vi "Thermistor_Callibration.vi"(11 "DataCluster in":T2={"Core"={"Current VI Reference"=refnum, "Close Panel on Exit?"=FALSE, "Exit"=FALSE, "Initialized?"=FALSE}, "Connections"={"cDAQ"={"Task"="", "Connected"=FALSE, "Active"=FALSE, "ID"=""}, "Camera"={"Session"="", "Connected"=FALSE, "Active"=FALSE, "Placeholder"=refnum}, "PSU"={"Port"="", "Connected"=FALSE, "Active"=FALSE}, "Arduino"={"Port"="", "Connected"=FALSE, "Active"=FALSE}}, "Data Acquisition"={"Setup"={"Label"="", "Operator"="", "Notes"="", "TempGrad"=1.0, "TargetTemp"=1.0, "Sample Volume"=1.0}, "Camera"={"Image"=refnum, "Save Image"=refnum, "Image Frequency"=20, "Rectangle"={"Left"=0, "Top"=0, "Right"=0, "Bottom"=0, "Rotation"=0.0}, "Calibration"={"Top Left"={"X"=0.0, "Y"=0.0}, "Top Right"={"X"=0.0, "Y"=0.0}, "Bottom Left"={"X"=0.0, "Y"=0.0}, "Bottom Right"={"X"=0.0, "Y"=0.0}, "Fixpoint"={"X"=0.0, "Y"=0.0}, "Scan Area"=0.0, "Fixpoint Area"=0.0, "Well Pixels"=[], "Valid"=FALSE}, "FocusPos"=0, "Display Mapping"=10, "Camera Mode"=10}, "Thermistor"={"Sample Size"=1, "Calibration"={"B0.100"=[], "R25"=[], "c"=[], "State"=[], "V_S"=5.0, "R_S"=100.0}, "Timing Mode"=14713}, "Partition"={"Data"=[], "Cell Label"="", "Cell Color"=0, "Height"=10, "Width"=16, "Grid"=[]}, "Queue"={"Size"=1, "Queue"=refnum}, "Sample Rate"=1, "Active"=FALSE, "Ready"=FALSE, "Graph Mode"=0, "Gradient Buffer"=2}, "Control"={"Sample Rate"=1, "PID gains"={"proportional gain (Kc)"=1.0, "integral time (Ti, min)"=0.01, "derivative time (Td, min)"=0.0}}, "Manual Temp Control"={"TargetTemp"=1.0, "Mode"=0, "Active"=FALSE}} {"Manual Temp Control"."Mode" items=["Cool", "Heat"]; "Manual Temp Control"."TargetTemp" min=-40.0 max=40.0 step=0.5 format="%#_g °C"; "Control"."PID gains"."derivative time (Td, min)" format="%.3f"; "Control"."PID gains"."integral time (Ti, min)" format="%.3f"; "Control"."PID gains"."proportional gain (Kc)" format="%.3f"; "Control"."Sample Rate" min=1 max=20 step=1 format="%.0f Samples/sec"; "Data Acquisition"."Gradient Buffer" min=2 max=30 step=1; "Data Acquisition"."Graph Mode" items=["Thermistor Temperature", "Camera Temperature"]; "Data Acquisition"."Thermistor"."Timing Mode" items=["Automatic"=16097, "High Resolution"=10195, "High Speed"=14712, "Best 50 Hz Rejection"=14713, "Best 60 Hz Rejection"=14714, "Custom"=10137]; "Data Acquisition"."Thermistor"."Calibration"."R_S" min=0.1 max=1000.0 format="%#_g kOhm"; "Data Acquisition"."Thermistor"."Calibration"."V_S" min=5.0 max=48.0 format="%#_g V"; "Data Acquisition"."Thermistor"."Calibration"."R25" min=0.1 max=1000.0 format="%#_g kOhm"; "Data Acquisition"."Thermistor"."Calibration"."B0.100" min=100.0 max=10000.0 format="%#_g K"; "Data Acquisition"."Thermistor"."Sample Size" min=1 max=200; "Data Acquisition"."Sample Rate" min=20 max=240 format="%.0f samples/min"; "Data Acquisition"."Queue"."Size" min=1 max=200; "Data Acquisition"."Camera"."Camera Mode" items=["Temperature Linear", "Signal Linear"]; "Data Acquisition"."Camera"."Display Mapping" items=["Default"=10, "Most Significant Bits"=11, "Full Dynamic"=12, "Downshift"=13, "Given Range"=14, "90% Dynamic"=15, "Given Percent Range"=16]; "Data Acquisition"."Camera"."Calibration"."Fixpoint"."Y" format="%.2f"; "Data Acquisition"."Camera"."Calibration"."Fixpoint"."X" format="%.2f"; "Data Acquisition"."Camera"."Calibration"."Top Left"."Y" format="%.2f"; "Data Acquisition"."Camera"."Calibration"."Top Left"."X" format="%.2f"; "Data Acquisition"."Camera"."Calibration"."Top Right"."Y" format="%.2f"; "Data Acquisition"."Camera"."Calibration"."Top Right"."X" format="%.2f"; "Data Acquisition"."Camera"."Calibration"."Bottom Left"."Y" format="%.2f"; "Data Acquisition"."Camera"."Calibration"."Bottom Left"."X" format="%.2f"; "Data Acquisition"."Camera"."Calibration"."Bottom Right"."Y" format="%.2f"; "Data Acquisition"."Camera"."Calibration"."Bottom Right"."X" format="%.2f"; "Data Acquisition"."Camera"."Rectangle"."Rotation" min=-90.0 max=90.0 step=1.0 format="%.2f"; "Data Acquisition"."Camera"."Rectangle"."Left" scale=0.0..1024.0; "Data Acquisition"."Camera"."Rectangle"."Right" scale=0.0..1024.0; "Data Acquisition"."Camera"."Image Frequency" min=1 max=60 step=1; "Data Acquisition"."Setup"."Sample Volume" min=0.0 max=500.0 format="%#_g µL"; "Data Acquisition"."Setup"."TargetTemp" min=-40.0 max=40.0 step=0.5 format="%#_g °C"; "Data Acquisition"."Setup"."TempGrad" min=-100.0 max=100.0 step=0.1 format="%#_g °C/min"}) -> (2 "State Out":string="Data: Save Calibration", 3 "DataCluster out":T2={"Core"={"Current VI Reference"=refnum, "Close Panel on Exit?"=FALSE, "Exit"=FALSE, "Initialized?"=FALSE}, "Connections"={"cDAQ"={"Task"="", "Connected"=FALSE, "Active"=FALSE, "ID"=""}, "Camera"={"Session"="", "Connected"=FALSE, "Active"=FALSE, "Placeholder"=refnum}, "PSU"={"Port"="", "Connected"=FALSE, "Active"=FALSE}, "Arduino"={"Port"="", "Connected"=FALSE, "Active"=FALSE}}, "Data Acquisition"={"Setup"={"Label"="", "Operator"="", "Notes"="", "TempGrad"=0.0, "TargetTemp"=0.0, "Sample Volume"=0.0}, "Camera"={"Image"=refnum, "Save Image"=refnum, "Image Frequency"=20, "Rectangle"={"Left"=0, "Top"=0, "Right"=0, "Bottom"=0, "Rotation"=0.0}, "Calibration"={"Top Left"={"X"=0.0, "Y"=0.0}, "Top Right"={"X"=0.0, "Y"=0.0}, "Bottom Left"={"X"=0.0, "Y"=0.0}, "Bottom Right"={"X"=0.0, "Y"=0.0}, "Fixpoint"={"X"=0.0, "Y"=0.0}, "Scan Area"=0.0, "Fixpoint Area"=0.0, "Well Pixels"=[], "Valid"=FALSE}, "FocusPos"=0, "Display Mapping"=10, "Camera Mode"=10}, "Thermistor"={"Sample Size"=0, "Calibration"={"B0.100"=[], "R25"=[], "c"=[], "State"=[], "V_S"=0.0, "R_S"=0.0}, "Timing Mode"=0}, "Partition"={"Data"=[], "Cell Label"="", "Cell Color"=0, "Height"=0, "Width"=0, "Grid"=[]}, "Queue"={"Size"=0, "Queue"=refnum}, "Sample Rate"=0, "Active"=FALSE, "Ready"=FALSE, "Graph Mode"=0, "Gradient Buffer"=2}, "Control"={"Sample Rate"=0, "PID gains"={"proportional gain (Kc)"=0.0, "integral time (Ti, min)"=0.0, "derivative time (Td, min)"=0.0}}, "Manual Temp Control"={"TargetTemp"=1.0, "Mode"=0, "Active"=FALSE}} {"Manual Temp Control"."Mode" items=["Cool", "Heat"]; "Manual Temp Control"."TargetTemp" min=-40.0 max=40.0 step=0.5 format="%#_g °C"; "Control"."PID gains"."derivative time (Td, min)" format="%.3f"; "Control"."PID gains"."integral time (Ti, min)" format="%.3f"; "Control"."PID gains"."proportional gain (Kc)" format="%.3f"; "Control"."Sample Rate" min=1 max=20 step=1 format="%.0f Samples/sec"; "Data Acquisition"."Gradient Buffer" min=2 max=30 step=1; "Data Acquisition"."Graph Mode" items=["Thermistor Temperature", "Camera Temperature"]; "Data Acquisition"."Thermistor"."Timing Mode" items=["Automatic"=16097, "High Resolution"=10195, "High Speed"=14712, "Best 50 Hz Rejection"=14713, "Best 60 Hz Rejection"=14714, "Custom"=10137]; "Data Acquisition"."Thermistor"."Calibration"."R_S" min=0.1 max=1000.0 format="%#_g kOhm"; "Data Acquisition"."Thermistor"."Calibration"."V_S" min=5.0 max=48.0 format="%#_g V"; "Data Acquisition"."Thermistor"."Calibration"."R25" min=0.1 max=1000.0 format="%#_g kOhm"; "Data Acquisition"."Thermistor"."Calibration"."B0.100" min=100.0 max=10000.0 format="%#_g K"; "Data Acquisition"."Thermistor"."Sample Size" min=1 max=200; "Data Acquisition"."Sample Rate" min=20 max=240 format="%.0f samples/min"; "Data Acquisition"."Queue"."Size" min=1 max=200; "Data Acquisition"."Camera"."Camera Mode" items=["Temperature Linear", "Signal Linear"]; "Data Acquisition"."Camera"."Display Mapping" items=["Default"=10, "Most Significant Bits"=11, "Full Dynamic"=12, "Downshift"=13, "Given Range"=14, "90% Dynamic"=15, "Given Percent Range"=16]; "Data Acquisition"."Camera"."Calibration"."Fixpoint"."Y" format="%.2f"; "Data Acquisition"."Camera"."Calibration"."Fixpoint"."X" format="%.2f"; "Data Acquisition"."Camera"."Calibration"."Top Left"."Y" format="%.2f"; "Data Acquisition"."Camera"."Calibration"."Top Left"."X" format="%.2f"; "Data Acquisition"."Camera"."Calibration"."Top Right"."Y" format="%.2f"; "Data Acquisition"."Camera"."Calibration"."Top Right"."X" format="%.2f"; "Data Acquisition"."Camera"."Calibration"."Bottom Left"."Y" format="%.2f"; "Data Acquisition"."Camera"."Calibration"."Bottom Left"."X" format="%.2f"; "Data Acquisition"."Camera"."Calibration"."Bottom Right"."Y" format="%.2f"; "Data Acquisition"."Camera"."Calibration"."Bottom Right"."X" format="%.2f"; "Data Acquisition"."Camera"."Rectangle"."Rotation" min=-90.0 max=90.0 step=1.0 format="%.2f"; "Data Acquisition"."Camera"."Rectangle"."Left" scale=0.0..1024.0; "Data Acquisition"."Camera"."Rectangle"."Right" scale=0.0..1024.0; "Data Acquisition"."Camera"."Image Frequency" min=1 max=60 step=1; "Data Acquisition"."Setup"."Sample Volume" min=0.0 max=500.0 format="%#_g µL"; "Data Acquisition"."Setup"."TargetTemp" min=-40.0 max=40.0 step=0.5 format="%#_g °C"; "Data Acquisition"."Setup"."TempGrad" min=-100.0 max=100.0 step=0.1 format="%#_g °C/min"})   [LabVIEW 2024]
uses:
  DataCluster.ctl
  <vilib>/userDefined/High Color/IMAQdx.ctl
  <vilib>/vision/Image Controls.llb/IMAQ Image.ctl
panel:
  in  "Ring":u16(ring) items=["Setup", "Thermistor (Ref.)", "Thermistor 1", "Thermistor 2", "Thermistor 3", "Thermistor 4", "Thermistor 5", "Thermistor 6"]
  out "Tab Control":T1(tab)
  in  "Supply Voltage":dbl=12.062 format="%#_g V"
  in  "Static Resistor":dbl=10.0 min=0.1 max=1000.0 format="%#_g kOhm"
  out "Active":bool
  in  "c ref":dbl[](array[numeric]) caption="constants" format="%_6g"
  in  "B0.100 ref":dbl caption="ß0.100" min=0.0 format="%#_g K"
  in  "R25 ref":dbl caption="R25" min=0.0 format="%#_g kOhm"
  in  "Active 1":bool
  in  "B0.100 1":dbl caption="ß0.100" min=0.0 format="%#_g K"
  in  "R25 1":dbl caption="R25" min=0.0 format="%#_g kOhm"
  in  "c 1":dbl[](array[numeric]) caption="constants" format="%_6g"
  in  "Active 2":bool
  in  "B0.100 2":dbl caption="ß0.100" min=0.0 format="%#_g K"
  in  "R25 2":dbl caption="R25" min=0.0 format="%#_g kOhm"
  in  "c 2":dbl[](array[numeric]) caption="constants" format="%_6g"
  in  "Active 3":bool
  in  "B0.100 3":dbl caption="ß0.100" min=0.0 format="%#_g K"
  in  "R25 3":dbl caption="R25" min=0.0 format="%#_g kOhm"
  in  "c 3":dbl[](array[numeric]) caption="constants" format="%_6g"
  in  "Active 4":bool
  in  "B0.100 4":dbl caption="ß0.100" min=0.0 format="%#_g K"
  in  "R25 4":dbl caption="R25" min=0.0 format="%#_g kOhm"
  in  "c 4":dbl[](array[numeric]) caption="constants" format="%_6g"
  in  "Active 5":bool
  in  "B0.100 5":dbl caption="ß0.100" min=0.0 format="%#_g K"
  in  "R25 5":dbl caption="R25" min=0.0 format="%#_g kOhm"
  in  "c 5":dbl[](array[numeric]) caption="constants" format="%_6g"
  in  "Active 6":bool
  in  "B0.100 6":dbl caption="ß0.100" min=0.0 format="%#_g K"
  in  "R25 6":dbl caption="R25" min=0.0 format="%#_g kOhm"
  in  "c 6":dbl[](array[numeric]) caption="constants" format="%_6g"
  in  "Cancel":bool
  in  "OK":bool
  # "Adjust thermistor calibration values used in conversion between measured voltages and temperatures"
  # "c0"
  # "c1"
  # "c2"
  # "c3"
  # "c4"
  # "c0"
  # "c1"
  # "c2"
  # "c3"
  # "c4"
  # "c0"
  # "c1"
  # "c2"
  # "c3"
  # "c4"
  # "c0"
  # "c1"
  # "c2"
  # "c3"
  # "c4"
  # "c0"
  # "c1"
  # "c2"
  # "c3"
  # "c4"
  # "c0"
  # "c1"
  # "c2"
  # "c3"
  # "c4"
  # "c0"
  # "c1"
  # "c2"
  # "c3"
  # "c4"
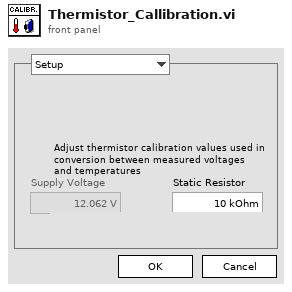
[diagram p1: front panel]
types:
  T1 = enum32{"Setup", "1", "2", "3", "4", "5", "6", "7", "8"}
  T2 = typedef "DataCluster.ctl" = cluster{"Core":cluster{"Current VI Reference":refnum<vi>, "Close Panel on Exit?":bool, "Exit":bool, "Initialized?":bool}, "Connections":cluster{"cDAQ":cluster{"Task":refnum<k21>, "Connected":bool, "Active":bool, "ID":string}, "Camera":cluster{"Session":T3, "Connected":bool, "Active":bool, "Placeholder":T4}, "PSU":cluster{"Port":refnum<visa-resource-name>, "Connected":bool, "Active":bool}, "Arduino":cluster{"Port":refnum<visa-resource-name>, "Connected":bool, "Active":bool}}, "Data Acquisition":cluster{"Setup":cluster{"Label":string, "Operator":string, "Notes":string, "TempGrad":dbl, "TargetTemp":dbl, "Sample Volume":dbl}, "Camera":cluster{"Image":T4, "Save Image":T4, "Image Frequency":i32, "Rectangle":T5, "Calibration":cluster{"Top Left":T6, "Top Right":T6, "Bottom Left":T6, "Bottom Right":T6, "Fixpoint":T6, "Scan Area":dbl, "Fixpoint Area":dbl, "Well Pixels":cluster{"X":i32, "Y":i32}[][], "Valid":bool}, "FocusPos":u32, "Display Mapping":u32, "Camera Mode":u32}, "Thermistor":cluster{"Sample Size":i32, "Calibration":cluster{"B0.100":dbl[], "R25":dbl[], "c":dbl[][], "State":bool[], "V_S":dbl, "R_S":dbl}, "Timing Mode":i32}, "Partition":cluster{"Data":string[][], "Cell Label":string, "Cell Color":u32, "Height":i32, "Width":i32, "Grid":string[][]}, "Queue":cluster{"Size":i32, "Queue":refnum<queue>}, "Sample Rate":i32, "Active":bool, "Ready":bool, "Graph Mode":u16, "Gradient Buffer":i32}, "Control":cluster{"Sample Rate":i32, "PID gains":cluster{"proportional gain (Kc)":dbl, "integral time (Ti, min)":dbl, "derivative time (Td, min)":dbl}}, "Manual Temp Control":cluster{"TargetTemp":dbl, "Mode":u16, "Active":bool}}
  T3 = typedef "IMAQdx.ctl" = refnum<k21>
  T4 = typedef "IMAQ Image.ctl" = refnum<image>
  T5 = typedef "IMAQ Rectangle" = cluster{"Left":i32, "Top":i32, "Right":i32, "Bottom":i32, "Rotation":dbl}
  T6 = typedef "IMAQ Point" = cluster{"X":sgl, "Y":sgl}
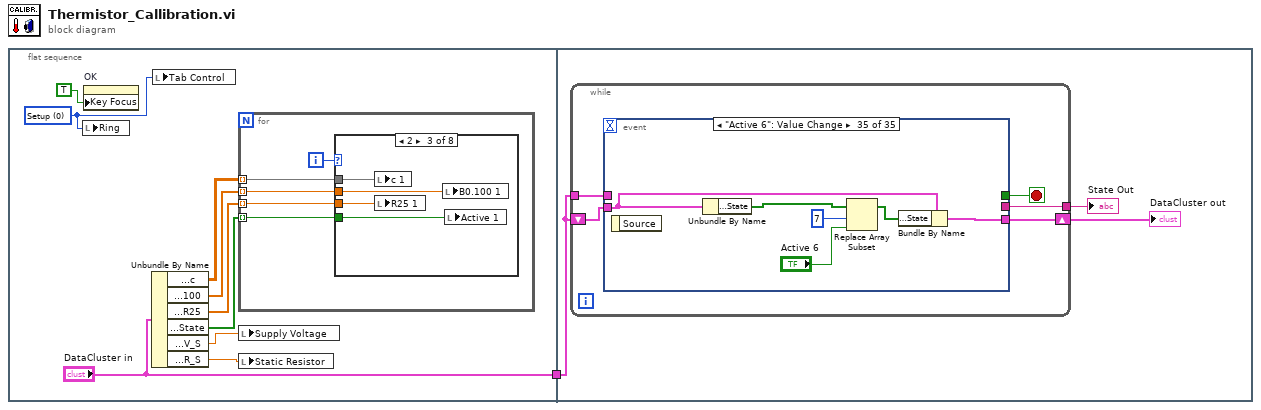
[diagram p0: block diagram]
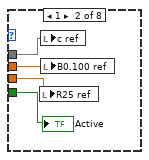
[diagram p3: hidden frame]
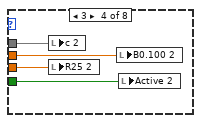
[diagram p4: hidden frame]
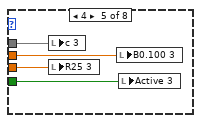
[diagram p5: hidden frame]
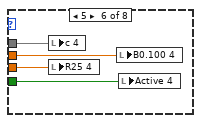
[diagram p6: hidden frame]
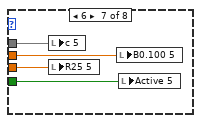
[diagram p7: hidden frame]
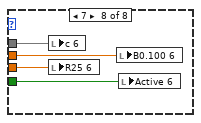
[diagram p8: hidden frame]
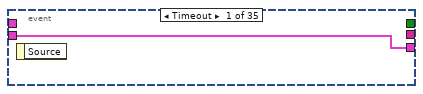
[diagram p9: hidden frame]
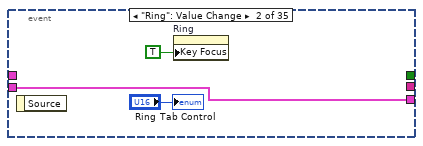
[diagram p10: hidden frame]
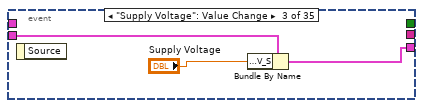
[diagram p11: hidden frame]
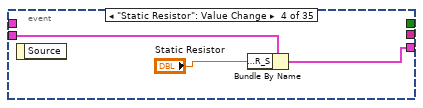
[diagram p12: hidden frame]
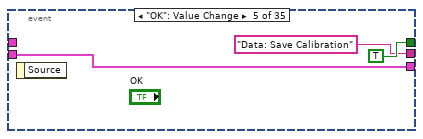
[diagram p13: hidden frame]
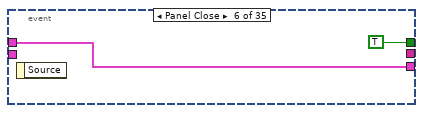
[diagram p14: hidden frame]
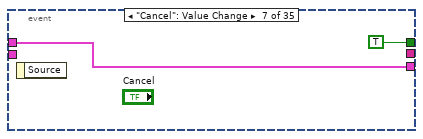
[diagram p15: hidden frame]
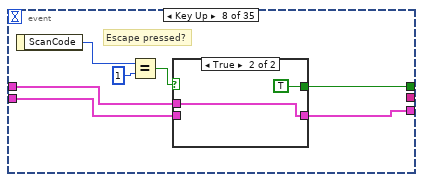
[diagram p16: hidden frame]
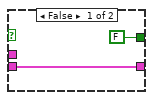
[diagram p17: hidden frame]
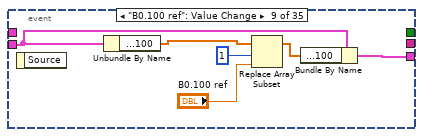
[diagram p18: hidden frame]
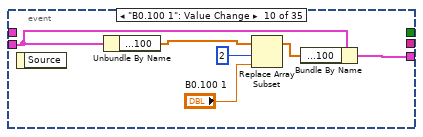
[diagram p19: hidden frame]
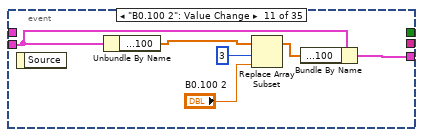
[diagram p20: hidden frame]
diagram:
  n1 = flat-sequence {
    tunnel: ["DataCluster in"] -> w1
    tunnel: w1 -> [w46]
    frame #0 {
      w4 = u16 0 items=["Setup", "Thermistor (Ref.)", "Thermistor 1", "Thermistor 2", "Thermistor 3", "Thermistor 4", "Thermistor 5", "Thermistor 6"] ("Ring")
      n2 = local write "Ring"(w4) -> ()
      n3 = property on="OK" class="Bool"("Key Focus"=TRUE) -> ()  [unwired: 2 in, 2 out]
      n4 = Unbundle By Name("DataCluster in") -> ("Data Acquisition.Thermistor.Calibration.c"=w3:dbl[][], "Data Acquisition.Thermistor.Calibration.B0.100"=w5:dbl[], "Data Acquisition.Thermistor.Calibration.R25"=w6:dbl[], "Data Acquisition.Thermistor.Calibration.State"=w2:bool[], "Data Acquisition.Thermistor.Calibration.V_S"=w8:dbl, "Data Acquisition.Thermistor.Calibration.R_S"=w7:dbl)
      n5 = local write "Tab Control"(w4) -> ()
      n6 = for {
        tunnel: w6 -> [w14] mode=indexing
        tunnel: w5 -> [w13] mode=indexing
        tunnel: w3 -> [w12] mode=indexing
        tunnel: w2 -> [w11] mode=indexing
        i -> [w15]
        n7 = case shown="2" w15 {
          tunnel: w14 -> [_ w19 w23 w27 w31 w35 w39 w43]
          tunnel: w13 -> [_ w18 w22 w26 w30 w34 w38 w42]
          tunnel: w12 -> [_ w17 w21 w25 w29 w33 w37 w41]
          tunnel: w11 -> [_ w16 w20 w24 w28 w32 w36 w40]
          frame 0, Default {
          }
          frame 1 {
            n8 = local write "R25 ref"(w19) -> ()
            n9 = local write "c ref"(w17) -> ()
            n10 = local write "B0.100 ref"(w18) -> ()
            "Active" <- w16
          }
          frame 2 {
            n11 = local write "c 1"(w21) -> ()
            n12 = local write "R25 1"(w23) -> ()
            n13 = local write "B0.100 1"(w22) -> ()
            n14 = local write "Active 1"(w20) -> ()
          }
          frame 3 {
            n15 = local write "c 2"(w25) -> ()
            n16 = local write "R25 2"(w27) -> ()
            n17 = local write "B0.100 2"(w26) -> ()
            n18 = local write "Active 2"(w24) -> ()
          }
          frame 4 {
            n19 = local write "c 3"(w29) -> ()
            n20 = local write "R25 3"(w31) -> ()
            n21 = local write "B0.100 3"(w30) -> ()
            n22 = local write "Active 3"(w28) -> ()
          }
          frame 5 {
            n23 = local write "c 4"(w33) -> ()
            n24 = local write "R25 4"(w35) -> ()
            n25 = local write "B0.100 4"(w34) -> ()
            n26 = local write "Active 4"(w32) -> ()
          }
          frame 6 {
            n27 = local write "c 5"(w37) -> ()
            n28 = local write "R25 5"(w39) -> ()
            n29 = local write "B0.100 5"(w38) -> ()
            n30 = local write "Active 5"(w36) -> ()
          }
          frame 7 {
            n31 = local write "c 6"(w41) -> ()
            n32 = local write "R25 6"(w43) -> ()
            n33 = local write "B0.100 6"(w42) -> ()
            n34 = local write "Active 6"(w40) -> ()
          }
        }
      }
      n35 = local write "Supply Voltage"(w8) -> ()
      n36 = local write "Static Resistor"(w7) -> ()
    }
    frame #1 {
      n37 = while {
        shift-right: [w51] -> w45
        shift-left: w46 -> [w50]
        tunnel: w46 -> [w49]
        tunnel: [w47] -> w44
        stop <- w48 stop-if-true
        n38 = event shown="[34] \"Active 6\": Value Change" {
          selector: _ -> [_ _ _ _ _ _ _ _ _ _ _ _ _ _ _ _ _ _ _ _ _ _ _ _ _ _ _ _ _ _ _ _ _ _ _]
          dyn-events: _ -> [_ _ _ _ _ _ _ _ _ _ _ _ _ _ _ _ _ _ _ _ _ _ _ _ _ _ _ _ _ _ _ _ _ _ _]
          timeout: _ -> [_ _ _ _ _ _ _ _ _ _ _ _ _ _ _ _ _ _ _ _ _ _ _ _ _ _ _ _ _ _ _ _ _ _ _]
          tunnel: w50 -> [w52 w54 w58 w61 w64 _ _ w69 w84 w90 w96 w102 w108 w114 w120 w126 w132 w138 w144 w150 w156 w162 w168 w174 w180 w186 w192 w198 w204 w210 w216 w222 w228 w234 w240]
          tunnel: [w52 w54 w57 w60 w64 w65 w68 w71 w85 w91 w97 w103 w109 w115 w121 w127 w133 w139 w145 w151 w157 w163 w169 w175 w181 w187 w193 w199 w205 w211 w217 w223 w229 w235 w241] -> w51
          tunnel: w49 -> [_ _ _ _ _ w65 w68 w70 _ _ _ _ _ _ _ _ _ _ _ _ _ _ _ _ _ _ _ _ _ _ _ _ _ _ _]
          tunnel: [_ _ _ _ TRUE TRUE TRUE w75 _ _ _ _ _ _ _ _ _ _ _ _ _ _ _ _ _ _ _ _ _ _ _ _ _ _ _] -> w48
          tunnel: [_ _ _ _ "Data: Save Calibration" _ _ _ _ _ _ _ _ _ _ _ _ _ _ _ _ _ _ _ _ _ _ _ _ _ _ _ _ _ _] -> w47
          event Timeout {
            n39 = event-data() -> ()  [unwired: 1 in, 1 out]
          }
          event "Ring": Value Change {
            n40 = event-data() -> ()  [unwired: 1 in, 1 out]
            n41 = property on="Ring" class="Ring (strict)"("Key Focus"=TRUE) -> ()  [unwired: 2 in, 2 out]
            "Tab Control" <- "Ring"
          }
          event "Supply Voltage": Value Change {
            n42 = event-data() -> ()  [unwired: 1 in, 1 out]
            n43 = Bundle By Name(cluster=w58, "Data Acquisition.Thermistor.Calibration.V_S"="Supply Voltage") -> (w57:T2)
          }
          event "Static Resistor": Value Change {
            n44 = event-data() -> ()  [unwired: 1 in, 1 out]
            n45 = Bundle By Name(cluster=w61, "Data Acquisition.Thermistor.Calibration.R_S"="Static Resistor") -> (w60:T2)
          }
          event "OK": Value Change {
            n46 = event-data() -> ()  [unwired: 1 in, 1 out]
          }
          event Panel Close {
            n47 = event-data() -> ()  [unwired: 1 in, 1 out]
          }
          event "Cancel": Value Change {
            n48 = event-data() -> ()  [unwired: 1 in, 1 out]
          }
          event Key Up {
            # "Escape pressed?"
            n49 = event-data() -> ("ScanCode"=w74:i16)  [unwired: 1 in]
            n50 = Equal?(x=w74, y=i16 1) -> (x = y?=w72:bool)
            n51 = case shown="True" w72 {
              tunnel: [FALSE TRUE] -> w75
              tunnel: [w77 w78] -> w71
              tunnel: w70 -> [_ w78]
              tunnel: w69 -> [w77 _]
              frame False {
              }
              frame True {
              }
            }
          }
          event "B0.100 ref": Value Change {
            n52 = event-data() -> ()  [unwired: 1 in, 1 out]
            n53 = Unbundle By Name(w84) -> ("Data Acquisition.Thermistor.Calibration.B0.100"=w83:dbl[])
            n54 = Replace Array Subset(array=w83, new element="B0.100 ref", index=1) -> (w80:dbl[])
            n55 = Bundle By Name(cluster=w84, "Data Acquisition.Thermistor.Calibration.B0.100"=w80) -> (w85:T2)
          }
          event "B0.100 1": Value Change {
            n56 = event-data() -> ()  [unwired: 1 in, 1 out]
            n57 = Unbundle By Name(w90) -> ("Data Acquisition.Thermistor.Calibration.B0.100"=w89:dbl[])
            n58 = Replace Array Subset(array=w89, new element="B0.100 1", index=2) -> (w87:dbl[])
            n59 = Bundle By Name(cluster=w90, "Data Acquisition.Thermistor.Calibration.B0.100"=w87) -> (w91:T2)
          }
          event "B0.100 2": Value Change {
            n60 = event-data() -> ()  [unwired: 1 in, 1 out]
            n61 = Unbundle By Name(w96) -> ("Data Acquisition.Thermistor.Calibration.B0.100"=w95:dbl[])
            n62 = Replace Array Subset(array=w95, new element="B0.100 2", index=3) -> (w93:dbl[])
            n63 = Bundle By Name(cluster=w96, "Data Acquisition.Thermistor.Calibration.B0.100"=w93) -> (w97:T2)
          }
          event "B0.100 3": Value Change {
            n64 = event-data() -> ()  [unwired: 1 in, 1 out]
            n65 = Unbundle By Name(w102) -> ("Data Acquisition.Thermistor.Calibration.B0.100"=w101:dbl[])
            n66 = Replace Array Subset(array=w101, new element="B0.100 3", index=4) -> (w99:dbl[])
            n67 = Bundle By Name(cluster=w102, "Data Acquisition.Thermistor.Calibration.B0.100"=w99) -> (w103:T2)
          }
          event "B0.100 4": Value Change {
            n68 = event-data() -> ()  [unwired: 1 in, 1 out]
            n69 = Unbundle By Name(w108) -> ("Data Acquisition.Thermistor.Calibration.B0.100"=w107:dbl[])
            n70 = Replace Array Subset(array=w107, new element="B0.100 4", index=5) -> (w105:dbl[])
            n71 = Bundle By Name(cluster=w108, "Data Acquisition.Thermistor.Calibration.B0.100"=w105) -> (w109:T2)
          }
          event "B0.100 5": Value Change {
            n72 = event-data() -> ()  [unwired: 1 in, 1 out]
            n73 = Unbundle By Name(w114) -> ("Data Acquisition.Thermistor.Calibration.B0.100"=w113:dbl[])
            n74 = Replace Array Subset(array=w113, new element="B0.100 5", index=6) -> (w111:dbl[])
            n75 = Bundle By Name(cluster=w114, "Data Acquisition.Thermistor.Calibration.B0.100"=w111) -> (w115:T2)
          }
          event "B0.100 6": Value Change {
            n76 = event-data() -> ()  [unwired: 1 in, 1 out]
            n77 = Unbundle By Name(w120) -> ("Data Acquisition.Thermistor.Calibration.B0.100"=w119:dbl[])
            n78 = Replace Array Subset(array=w119, new element="B0.100 6", index=7) -> (w117:dbl[])
            n79 = Bundle By Name(cluster=w120, "Data Acquisition.Thermistor.Calibration.B0.100"=w117) -> (w121:T2)
          }
          event "R25 ref": Value Change {
            n80 = event-data() -> ()  [unwired: 1 in, 1 out]
            n81 = Unbundle By Name(w126) -> ("Data Acquisition.Thermistor.Calibration.R25"=w125:dbl[])
            n82 = Replace Array Subset(array=w125, new element="R25 ref", index=1) -> (w123:dbl[])
            n83 = Bundle By Name(cluster=w126, "Data Acquisition.Thermistor.Calibration.R25"=w123) -> (w127:T2)
          }
          event "R25 1": Value Change {
            n84 = event-data() -> ()  [unwired: 1 in, 1 out]
            n85 = Unbundle By Name(w132) -> ("Data Acquisition.Thermistor.Calibration.R25"=w131:dbl[])
            n86 = Replace Array Subset(array=w131, new element="R25 1", index=2) -> (w129:dbl[])
            n87 = Bundle By Name(cluster=w132, "Data Acquisition.Thermistor.Calibration.R25"=w129) -> (w133:T2)
          }
          event "R25 2": Value Change {
            n88 = event-data() -> ()  [unwired: 1 in, 1 out]
            n89 = Unbundle By Name(w138) -> ("Data Acquisition.Thermistor.Calibration.R25"=w137:dbl[])
            n90 = Replace Array Subset(array=w137, new element="R25 2", index=3) -> (w135:dbl[])
            n91 = Bundle By Name(cluster=w138, "Data Acquisition.Thermistor.Calibration.R25"=w135) -> (w139:T2)
          }
          event "R25 3": Value Change {
            n92 = event-data() -> ()  [unwired: 1 in, 1 out]
            n93 = Unbundle By Name(w144) -> ("Data Acquisition.Thermistor.Calibration.R25"=w143:dbl[])
            n94 = Replace Array Subset(array=w143, new element="R25 3", index=4) -> (w141:dbl[])
            n95 = Bundle By Name(cluster=w144, "Data Acquisition.Thermistor.Calibration.R25"=w141) -> (w145:T2)
          }
          event "R25 4": Value Change {
            n96 = event-data() -> ()  [unwired: 1 in, 1 out]
            n97 = Unbundle By Name(w150) -> ("Data Acquisition.Thermistor.Calibration.R25"=w149:dbl[])
            n98 = Replace Array Subset(array=w149, new element="R25 4", index=5) -> (w147:dbl[])
            n99 = Bundle By Name(cluster=w150, "Data Acquisition.Thermistor.Calibration.R25"=w147) -> (w151:T2)
          }
          event "R25 5": Value Change {
            n100 = event-data() -> ()  [unwired: 1 in, 1 out]
            n101 = Unbundle By Name(w156) -> ("Data Acquisition.Thermistor.Calibration.R25"=w155:dbl[])
            n102 = Replace Array Subset(array=w155, new element="R25 5", index=6) -> (w153:dbl[])
            n103 = Bundle By Name(cluster=w156, "Data Acquisition.Thermistor.Calibration.R25"=w153) -> (w157:T2)
          }
          event "R25 6": Value Change {
            n104 = event-data() -> ()  [unwired: 1 in, 1 out]
            n105 = Unbundle By Name(w162) -> ("Data Acquisition.Thermistor.Calibration.R25"=w161:dbl[])
            n106 = Replace Array Subset(array=w161, new element="R25 6", index=7) -> (w159:dbl[])
            n107 = Bundle By Name(cluster=w162, "Data Acquisition.Thermistor.Calibration.R25"=w159) -> (w163:T2)
          }
          event "c ref": Value Change {
            n108 = event-data() -> ()  [unwired: 1 in, 1 out]
            n109 = Unbundle By Name(w168) -> ("Data Acquisition.Thermistor.Calibration.c"=w167:dbl[][])
            n110 = Replace Array Subset(array=w167, new element="c ref", index (row)=1 ("index")) -> (w165:dbl[][])  [unwired: 1 in]
            n111 = Bundle By Name(cluster=w168, "Data Acquisition.Thermistor.Calibration.c"=w165) -> (w169:T2)
          }
          event "c 1": Value Change {
            n112 = event-data() -> ()  [unwired: 1 in, 1 out]
            n113 = Unbundle By Name(w174) -> ("Data Acquisition.Thermistor.Calibration.c"=w173:dbl[][])
            n114 = Replace Array Subset(array=w173, new element="c 1", index (row)=2 ("index")) -> (w171:dbl[][])  [unwired: 1 in]
            n115 = Bundle By Name(cluster=w174, "Data Acquisition.Thermistor.Calibration.c"=w171) -> (w175:T2)
          }
          event "c 2": Value Change {
            n116 = event-data() -> ()  [unwired: 1 in, 1 out]
            n117 = Unbundle By Name(w180) -> ("Data Acquisition.Thermistor.Calibration.c"=w179:dbl[][])
            n118 = Replace Array Subset(array=w179, new element="c 2", index (row)=3 ("index")) -> (w177:dbl[][])  [unwired: 1 in]
            n119 = Bundle By Name(cluster=w180, "Data Acquisition.Thermistor.Calibration.c"=w177) -> (w181:T2)
          }
          event "c 3": Value Change {
            n120 = event-data() -> ()  [unwired: 1 in, 1 out]
            n121 = Unbundle By Name(w186) -> ("Data Acquisition.Thermistor.Calibration.c"=w185:dbl[][])
            n122 = Replace Array Subset(array=w185, new element="c 3", index (row)=4 ("index")) -> (w183:dbl[][])  [unwired: 1 in]
            n123 = Bundle By Name(cluster=w186, "Data Acquisition.Thermistor.Calibration.c"=w183) -> (w187:T2)
          }
          event "c 4": Value Change {
            n124 = event-data() -> ()  [unwired: 1 in, 1 out]
            n125 = Unbundle By Name(w192) -> ("Data Acquisition.Thermistor.Calibration.c"=w191:dbl[][])
            n126 = Replace Array Subset(array=w191, new element="c 4", index (row)=5 ("index")) -> (w189:dbl[][])  [unwired: 1 in]
            n127 = Bundle By Name(cluster=w192, "Data Acquisition.Thermistor.Calibration.c"=w189) -> (w193:T2)
          }
          event "c 5": Value Change {
            n128 = event-data() -> ()  [unwired: 1 in, 1 out]
            n129 = Unbundle By Name(w198) -> ("Data Acquisition.Thermistor.Calibration.c"=w197:dbl[][])
            n130 = Replace Array Subset(array=w197, new element="c 5", index (row)=6 ("index")) -> (w195:dbl[][])  [unwired: 1 in]
            n131 = Bundle By Name(cluster=w198, "Data Acquisition.Thermistor.Calibration.c"=w195) -> (w199:T2)
          }
          event "c 6": Value Change {
            n132 = event-data() -> ()  [unwired: 1 in, 1 out]
            n133 = Unbundle By Name(w204) -> ("Data Acquisition.Thermistor.Calibration.c"=w203:dbl[][])
            n134 = Replace Array Subset(array=w203, new element="c 6", index (row)=7 ("index")) -> (w201:dbl[][])  [unwired: 1 in]
            n135 = Bundle By Name(cluster=w204, "Data Acquisition.Thermistor.Calibration.c"=w201) -> (w205:T2)
          }
          event "Active 1": Value Change {
            n136 = event-data() -> ()  [unwired: 1 in, 1 out]
            n137 = Unbundle By Name(w210) -> ("Data Acquisition.Thermistor.Calibration.State"=w209:bool[])
            n138 = Replace Array Subset(array=w209, new element="Active 1", index=2) -> (w207:bool[])
            n139 = Bundle By Name(cluster=w210, "Data Acquisition.Thermistor.Calibration.State"=w207) -> (w211:T2)
          }
          event "Active 2": Value Change {
            n140 = event-data() -> ()  [unwired: 1 in, 1 out]
            n141 = Unbundle By Name(w216) -> ("Data Acquisition.Thermistor.Calibration.State"=w215:bool[])
            n142 = Replace Array Subset(array=w215, new element="Active 2", index=3) -> (w213:bool[])
            n143 = Bundle By Name(cluster=w216, "Data Acquisition.Thermistor.Calibration.State"=w213) -> (w217:T2)
          }
          event "Active 3": Value Change {
            n144 = event-data() -> ()  [unwired: 1 in, 1 out]
            n145 = Unbundle By Name(w222) -> ("Data Acquisition.Thermistor.Calibration.State"=w221:bool[])
            n146 = Replace Array Subset(array=w221, new element="Active 3", index=4) -> (w219:bool[])
            n147 = Bundle By Name(cluster=w222, "Data Acquisition.Thermistor.Calibration.State"=w219) -> (w223:T2)
          }
          event "Active 4": Value Change {
            n148 = event-data() -> ()  [unwired: 1 in, 1 out]
            n149 = Unbundle By Name(w228) -> ("Data Acquisition.Thermistor.Calibration.State"=w227:bool[])
            n150 = Replace Array Subset(array=w227, new element="Active 4", index=5) -> (w225:bool[])
            n151 = Bundle By Name(cluster=w228, "Data Acquisition.Thermistor.Calibration.State"=w225) -> (w229:T2)
          }
          event "Active 5": Value Change {
            n152 = event-data() -> ()  [unwired: 1 in, 1 out]
            n153 = Unbundle By Name(w234) -> ("Data Acquisition.Thermistor.Calibration.State"=w233:bool[])
            n154 = Replace Array Subset(array=w233, new element="Active 5", index=6) -> (w231:bool[])
            n155 = Bundle By Name(cluster=w234, "Data Acquisition.Thermistor.Calibration.State"=w231) -> (w235:T2)
          }
          event "Active 6": Value Change {
            n156 = event-data() -> ()  [unwired: 1 in, 1 out]
            n157 = Unbundle By Name(w240) -> ("Data Acquisition.Thermistor.Calibration.State"=w239:bool[])
            n158 = Replace Array Subset(array=w239, new element="Active 6", index=7) -> (w237:bool[])
            n159 = Bundle By Name(cluster=w240, "Data Acquisition.Thermistor.Calibration.State"=w237) -> (w241:T2)
          }
        }
      }
      "DataCluster out" <- w45
      "State Out" <- w44
    }
  }
